vi "MeasuredObj_get.vi"(8 "error in (no error)":errorcluster) -> (0 "error out":errorcluster, 3 "MeasuredObjects":T1(array[cluster]))   [LabVIEW 2009, in "NetworkVarTarget.lvlib"]
uses:
  NetworkVarTarget.lvlib
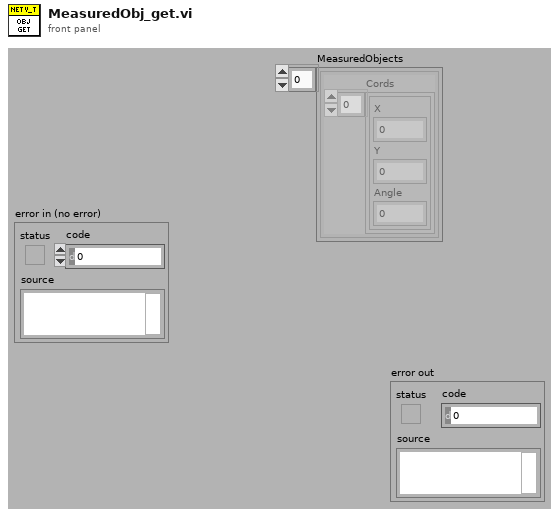
[diagram p1: front panel]
types:
  T1 = cluster{"Cords":cluster{"X":dbl, "Y":dbl, "Angle":dbl}[]}[]
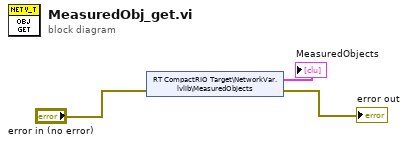
[diagram p0: block diagram]
diagram:
  n1 = shared-variable "RT CompactRIO Target\\NetworkVar.lvlib\\MeasuredObjects"(error in="error in (no error)") -> (→"MeasuredObjects":T1, error out=→"error out":errorcluster)
